vi "test Get-Set-Get Device Parameters.vi"(8 "error in":errorcluster, 11 "TestCase in":refnum<class "Scripting.lvclass">) -> (0 "error out":errorcluster, 3 "TestCase out":refnum<class "Scripting.lvclass">)   [LabVIEW 2020, in "Scripting.lvclass"]
uses:
  Scripting.lvclass
  <vilib>/addons/_JKI Toolkits/VI Tester/TestCase.llb/TestCase.lvclass
  Scripting/Ballard ARINC 429 Scripting.lvlib
  Shared/Initialization Method.ctl
  Shared/Device Parameters.ctl
  C:/Program Files (x86)/National Instruments/LabVIEW 2020/vi.lib/addons/_JKI Toolkits/VI Tester/TestCase.llb/TestCase.lvclass
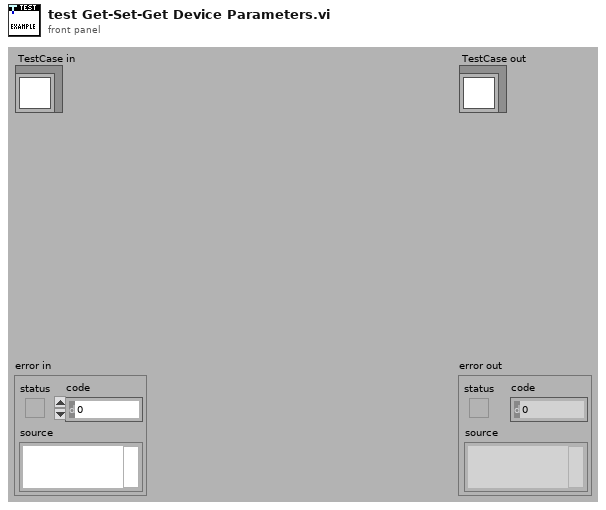
[diagram p1: front panel]
types:
  T1 = typedef "Device Parameters.ctl" = cluster{"initialization method":T2, "card number":i32, "PXI slot number":i32, "core number":i32}
  T2 = typedef "Initialization Method.ctl" = enum16{"PXI Slot Number", "Card Number"}
  T3 = typedef "Custom Device API.lvlib/Custom Device Item Ref.ctl" = u64
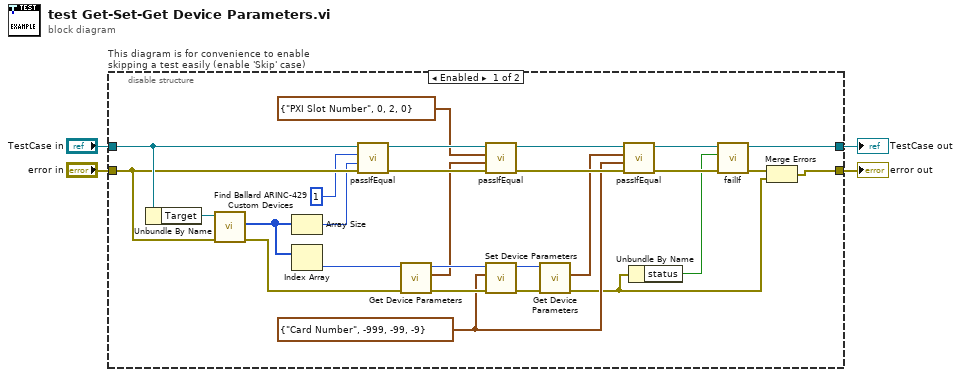
[diagram p0: block diagram]
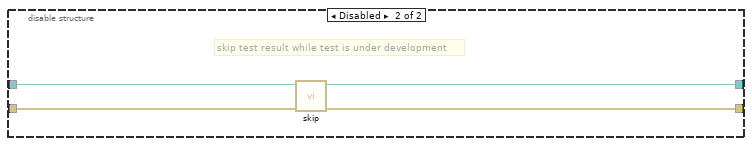
[diagram p2: hidden frame]
diagram:
  n1 = disable-structure "This diagram is for convenience to enable skipping a test easily (enable 'Skip' case)" shown="Enabled" {
    disable-tunnel: "TestCase in" -> [w30 w35]
    disable-tunnel: [w18 w33] -> w1
    disable-tunnel: [w26 w34] -> w3
    disable-tunnel: "error in" -> [w29 w32]
    frame Enabled {
      w10 = T1 {"initialization method"=enum."Card Number", "card number"=-999, "PXI slot number"=-99, "core number"=-9} ("device parameters")
      n2 = Unbundle By Name(w30) -> ("Target"=w31:refnum<k24>)
      n3 = call "Find Ballard ARINC-429 Custom Devices.vi"("error in"=w29, "target in"=w31) -> ("error out"=w16:errorcluster, "Ballard ARINC 429 custom devices"=w5:u64[])  [unwired: 7 in, 1 out]
      n4 = Array Size(array=w5) -> (size(s)=w27:i32)
      n5 = Index Array(array=w5) -> (element=w17:u64)  [unwired: 1 in]
      n6 = call-dynamic "passIfEqual.vi"("error in (no error)"=w29, "y"=w27, "x"=1 ("size(s)"), "TestCase in"=w30) -> ("error out"=w24:errorcluster, "TestCase out"=w25:refnum<class "Scripting.lvclass">)  [unwired: 6 in]
      n7 = call "Get Device Parameters.vi"("error in"=w16, "Ballard ARINC 429 custom device in"=w17) -> ("error out"=w14:errorcluster, "device parameters"=w9:T1, "Ballard ARINC 429 custom device out"=w15:T3)  [unwired: 7 in]
      n8 = call-dynamic "passIfEqual.vi"("error in (no error)"=w24, "y"=w9, "x"=T1 {"initialization method"=enum."PXI Slot Number", "card number"=0, "PXI slot number"=2, "core number"=0} ("device parameters"), "TestCase in"=w25) -> ("error out"=w22:errorcluster, "TestCase out"=w23:refnum<class "Scripting.lvclass">)  [unwired: 6 in]
      n9 = call "Set Device Parameters.vi"("error in"=w14, "device parameters"=w10, "Ballard ARINC 429 custom device in"=w15) -> ("error out"=w12:errorcluster, "Ballard ARINC 429 custom device out"=w13:T3)  [unwired: 7 in]
      n10 = call "Get Device Parameters.vi"("error in"=w12, "Ballard ARINC 429 custom device in"=w13) -> ("error out"=w7:errorcluster, "device parameters"=w11:T1)  [unwired: 7 in, 1 out]
      n11 = call-dynamic "passIfEqual.vi"("error in (no error)"=w22, "y"=w10, "x"=w11, "TestCase in"=w23) -> ("error out"=w20:errorcluster, "TestCase out"=w19:refnum<class "Scripting.lvclass">)  [unwired: 6 in]
      n12 = Unbundle By Name(w7) -> ("status"=w8:bool)
      n13 = call-dynamic "failIf.vi"("error in (no error)"=w20, "fail"=w8, "TestCase in"=w19) -> ("error out"=w21:errorcluster, "TestCase out"=w18:refnum<class "Scripting.lvclass">)  [unwired: 7 in]
      n14 = Merge Errors(w21, w7) -> (w26:errorcluster)
    }
    frame Disabled {
      # "skip test result while test is under development"
      n15 = call <vilib>:"skip.vi"("error in (no error)"=w32, "TestCase in"=w35) -> ("error out"=w34:errorcluster, "TestCase out"=w33:refnum<class "Scripting.lvclass">)  [unwired: 8 in]
    }
  }
  "error out" <- w3
  "TestCase out" <- w1
